vi "MediaMobile.vi"(0 "Tempi Fronti":i32[](array[numeric]), 2 "lenght Media":i32=12) -> (7 "Tempi medi":dbl[](array[numeric]))   [LabVIEW 2017]
uses:
  <vilib>/Analysis/baseanly.llb/Mean (DBL).vi
  <vilib>/Analysis/NI_AALBase.lvlib
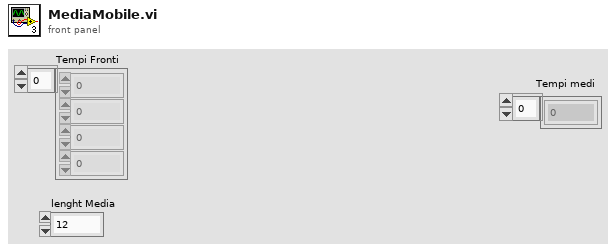
[diagram p1: front panel]
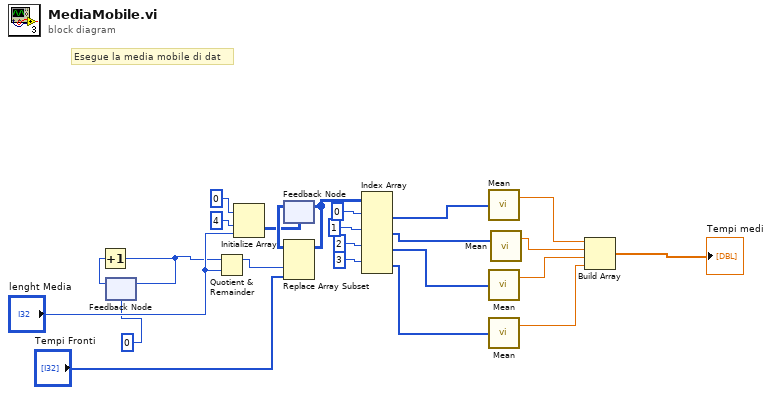
[diagram p0: block diagram]
diagram:
  # "Esegue la media mobile di dat"
  n1 = feedback #1(0) -> (w2:i32)
  n2 = Increment(x=w2) -> (x+1=w1:i32)
  n3 = feedback-in #1(w1) -> ()
  n4 = Quotient & Remainder(x=w1, y="lenght Media") -> (x-y*floor(x/y)=w4:i32)  [unwired: 1 out]
  n5 = Initialize Array(0, 4 ("dimension size"), "lenght Media") -> (w23:i32[][])
  n6 = feedback #2(w23) -> (w24:i32[][])
  n7 = Replace Array Subset(array=w24, new element="Tempi Fronti", index (col)=w4) -> (w19:i32[][])  [unwired: 1 in]
  n8 = feedback-in #2(w19) -> ()
  n9 = Index Array(array=w19, index (row) #1=0 ("index (row)"), index (row) #2=1 ("index (row)"), index (row) #3=2 ("index (row)"), index (row) #4=3 ("index (row)")) -> (element #1=w14:i32[], element #2=w13:i32[], element #3=w12:i32[], element #4=w11:i32[])  [unwired: 4 in]
  n10 = call-poly <vilib>:"Mean.vi"("X"=w14) -> ("mean"=w10:dbl)  [unwired: 1 out]
  n11 = call-poly <vilib>:"Mean.vi"("X"=w12) -> ("mean"=w8:dbl)  [unwired: 1 out]
  n12 = call-poly <vilib>:"Mean.vi"("X"=w11) -> ("mean"=w7:dbl)  [unwired: 1 out]
  n13 = call-poly <vilib>:"Mean.vi"("X"=w13) -> ("mean"=w9:dbl)  [unwired: 1 out]
  n14 = Build Array(w10, w9, w8, w7) -> (→"Tempi medi":dbl[])
